vi "MTS_GenFileComment.vi"(5 "Parent File No":i32=-1, 6 "Time Per Pixel [ms]":dbl, 7 "Measurement Type":T2(ring)=enum."Image File", 8 "error in":errorcluster, 9 "Upper Left":T4, 10 "Pixels":i32[](array[numeric]), 11 "Picture Size":dbl[](array[numeric])) -> (0 "error out":errorcluster, 1 "Image Header":T1, 2 "Image Info":T3, 3 "Comment":string)   [LabVIEW 2010]
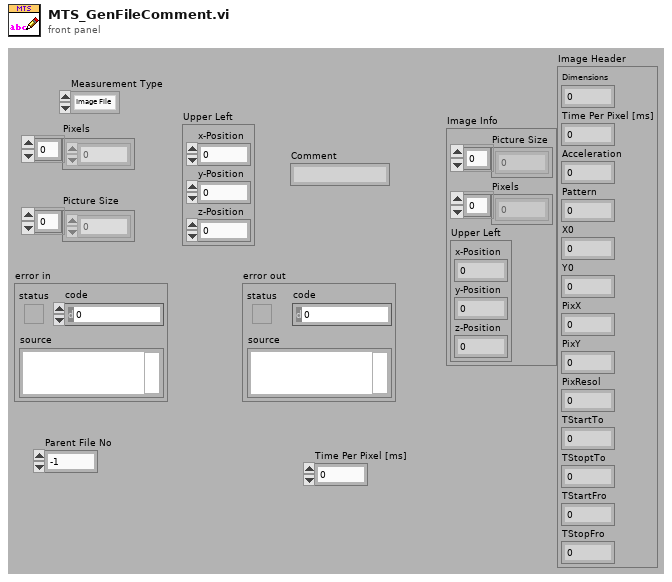
[diagram p1: front panel]
types:
  T1 = cluster{"Dimensions":i32, "Time Per Pixel [ms]":dbl, "Acceleration":i32, "Pattern":i32, "X0":sgl, "Y0":sgl, "PixX":i32, "PixY":i32, "PixResol":sgl, "TStartTo":sgl, "TStoptTo":sgl, "TStartFro":sgl, "TStopFro":sgl}
  T2 = enum16{"not a pt3 File", "Image File", "Point Measurement", "Auto Point"}
  T3 = cluster{"Picture Size":dbl[], "Pixels":i32[], "Upper Left":cluster{"x-Position":dbl, "y-Position":dbl, "z-Position":dbl}}
  T4 = cluster{"x-Position":dbl, "y-Position":dbl, "z-Position":dbl}
  T5 = cluster{"File No":i32, "File Path":path, "Parent File":i32, "File Type":enum16{"unknown", "pt3 File", "png Image", "bmp Image"}, "Measurement Type":enum16{"not a pt3 File", "Image File", "Point Measurement", "Auto Point"}, "Upper Left":cluster{"x-Position":dbl, "y-Position":dbl, "z-Position":dbl}, "Pixels":i32[], "Picture Size":dbl[], "Scan Axis":enum32{"x-y", "x-z", "y-z"}}
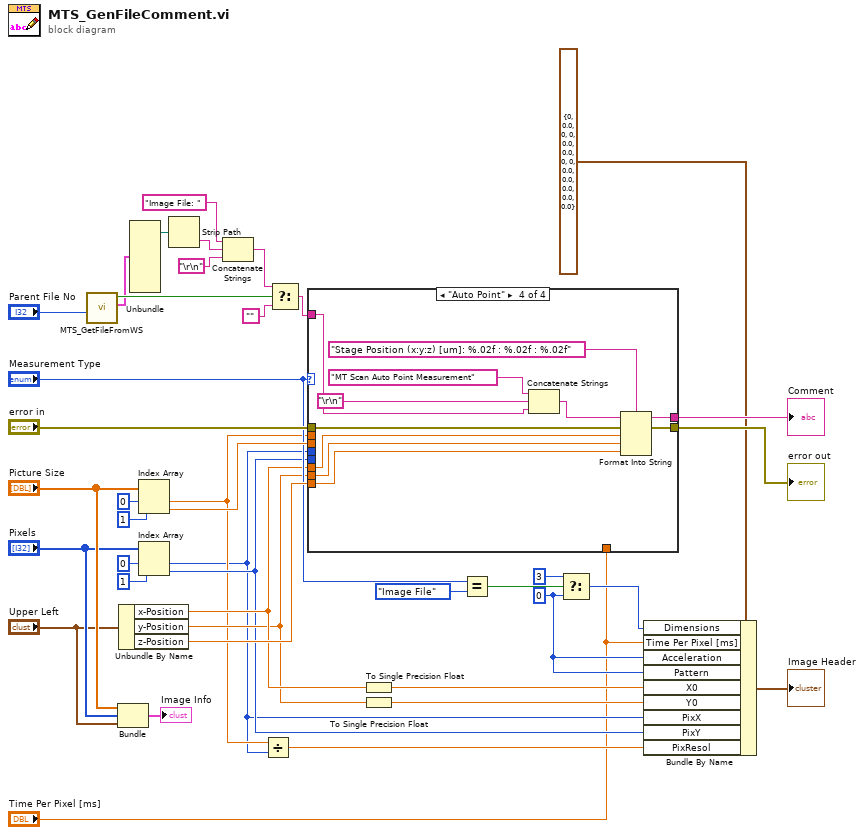
[diagram p0: block diagram]
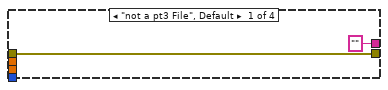
[diagram p2: hidden frame]
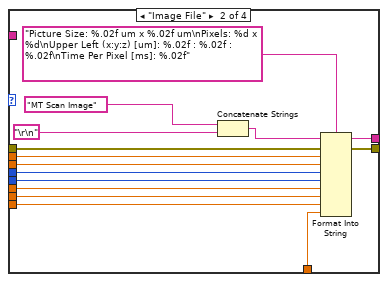
[diagram p3: hidden frame]
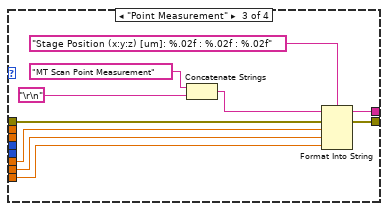
[diagram p4: hidden frame]
diagram:
  w20 = 0 ("f")
  n1 = call "MTS_GetFileFromWS.vi"("File No"="Parent File No") -> ("File Header"=w5:T5, "File Found"=w9:bool)  [unwired: 9 in]
  n2 = Bundle("Picture Size"="Picture Size", "Pixels"="Pixels", "Upper Left"="Upper Left") -> (→"Image Info":T3)  [unwired: 1 out]
  n3 = Unbundle By Name("Upper Left") -> ("x-Position"=w19:dbl, "y-Position"=w18:dbl, "z-Position"=w33:dbl)
  n4 = Unbundle(w5) -> ("File Path"=w4:path)  [unwired: 8 out]
  n5 = Index Array(array="Picture Size", index #1=0 ("index"), index #2=1 ("index")) -> (element #1=w14:dbl, element #2=w34:dbl)
  n6 = Index Array(array="Pixels", index #1=0 ("index"), index #2=1 ("index")) -> (element #1=w13:i32, element #2=w15:i32)
  n7 = Strip Path(path=w4) -> (name=w2:string)  [unwired: 1 out]
  n8 = Concatenate Strings("Image File: " ("string"), w2, "\r\n") -> (w3:string)
  n9 = Divide(x=w14, y=w13) -> (x/y=w12:dbl)
  n10 = Select(t=w3, s=w9, f="") -> (s? t:f=w7:string)
  n11 = case shown="\"Auto Point\"" "Measurement Type" {
    tunnel: [w42 w56 w66 w77] -> w40
    tunnel: "error in" -> [w42 w55 w65 w76]
    tunnel: w14 -> [_ w54 _ _]
    tunnel: w34 -> [_ w53 _ _]
    tunnel: w13 -> [_ w52 _ _]
    tunnel: w15 -> [_ w51 _ _]
    tunnel: w19 -> [_ w50 w63 w74]
    tunnel: w18 -> [_ w49 w62 w73]
    tunnel: w33 -> [_ w48 w61 w72]
    tunnel: ["" w47 w64 w75] -> w32
    tunnel: "Time Per Pixel [ms]" -> [_ w43 _ _]
    tunnel: w7 -> [_ _ _ w68]
    frame "not a pt3 File", Default {
    }
    frame "Image File" {
      n12 = Concatenate Strings("MT Scan Image" ("initial string"), "\r\n") -> (w44:string)
      n13 = Format Into String(format string="Picture Size: %.02f um x %.02f um\nPixels: %d x %d\nUpper Left (x:y:z) [um]: %.02f : %.02f : %.02f\nTime Per Pixel [ms]: %.02f", initial string=w44, error in=w55, w54, w53, w52, w51, w50, w49, w48, w43) -> (resulting string=w47:string, error out=w56:errorcluster)
    }
    frame "Point Measurement" {
      n14 = Concatenate Strings("MT Scan Point Measurement" ("initial string"), "\r\n") -> (w58:string)
      n15 = Format Into String(format string="Stage Position (x:y:z) [um]: %.02f : %.02f : %.02f", initial string=w58, error in=w65, w63, w62, w61) -> (resulting string=w64:string, error out=w66:errorcluster)
    }
    frame "Auto Point" {
      n16 = Concatenate Strings("MT Scan Auto Point Measurement" ("initial string"), "\r\n", w68) -> (w69:string)
      n17 = Format Into String(format string="Stage Position (x:y:z) [um]: %.02f : %.02f : %.02f", initial string=w69, error in=w76, w74, w73, w72) -> (resulting string=w75:string, error out=w77:errorcluster)
    }
  }
  "error out" <- w40
  "Comment" <- w32
  n18 = To Single Precision Float(number=w19) -> (single precision float=w17:sgl)
  n19 = To Single Precision Float(number=w18) -> (single precision float=w16:sgl)
  n20 = Equal?(x="Measurement Type", y=T2."Image File") -> (x = y?=w23:bool)
  n21 = Select(t=3, s=w23, f=w20) -> (s? t:f=w21:i32)
  n22 = Bundle By Name(cluster=T1 {"Dimensions"=0, "Time Per Pixel [ms]"=0.0, "Acceleration"=0, "Pattern"=0, "X0"=0.0, "Y0"=0.0, "PixX"=0, "PixY"=0, "PixResol"=0.0, "TStartTo"=0.0, "TStoptTo"=0.0, "TStartFro"=0.0, "TStopFro"=0.0} ("Image Header"), "Dimensions"=w21, "Time Per Pixel [ms]"="Time Per Pixel [ms]", "Acceleration"=w20, "Pattern"=w20, "X0"=w17, "Y0"=w16, "PixX"=w13, "PixY"=w15, "PixResol"=w12) -> (→"Image Header":T1)
